vi "LabVIEW time to Unix.vi"(1 "LabVIEW time":i64) -> (0 "Unix time":i64)   [LabVIEW 2018]
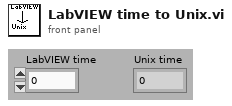
[diagram p1: front panel]
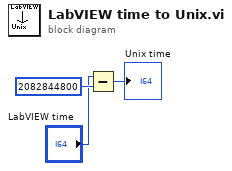
[diagram p0: block diagram]
diagram:
  n1 = Subtract(x="LabVIEW time", y=i64 2082844800) -> (x-y=→"Unix time":i64)
